vi "ClusterWithEnum.vi"(11 "Cluster":T1) -> ()   [LabVIEW 2013]
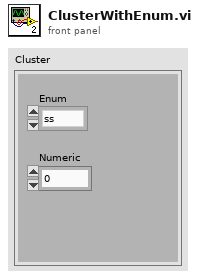
[diagram p1: front panel]
types:
  T1 = cluster{"Enum":enum16{"ss", "mm", "hh"}, "Numeric":dbl}
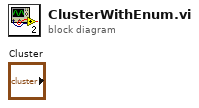
[diagram p0: block diagram]
diagram:
